vi "Reset hour counter.vi"(8 "error in (no error)":errorcluster, 10 "Button - Reset hour counter":bool, 11 "Frame Signal Conversion in":refnum<class "Frame Signal Conversion.lvclass">) -> (0 "error out":errorcluster, 3 "Frame Signal Conversion out":refnum<class "Frame Signal Conversion.lvclass">)   [LabVIEW 2024]
uses:
  Frame Signal Conversion Version 8 2015/Frame Signal Conversion Version 8/Frame Signal Conversion.lvclass
  <instrlib>/KDI Digital Instrumentation/API_for_PCAN_BASIC_FD/TPCANHandle.ctl
  Frame Signal Conversion Version 8 2015/Frame Signal Conversion Version 8/Signals to Frames/Convert Signals to Frames [Doubles].vi
  ZeroJet Test Systems/Instruments/PCAN/Polymorphic/DBC frame array to PCAN frame array.vi
  ZeroJet Test Systems/Instruments/PCAN/PCan_Xnet.lvlib
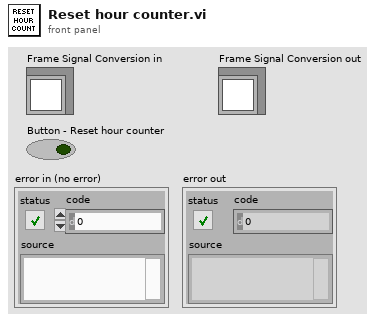
[diagram p1: front panel]
types:
  T1 = typedef "TPCANHandle.ctl" = enum16{"PCAN_NONEBUS  0x000", "PCAN_ISABUS1  0x21", "PCAN_ISABUS2  0x22", "PCAN_ISABUS3  0x23", "PCAN_ISABUS4  0x24", "PCAN_ISABUS5  0x25", "PCAN_ISABUS6  0x26", "PCAN_ISABUS7  0x27", "PCAN_ISABUS8  0x28", "PCAN_DNGBUS1  0x31", "PCAN_PCIBUS1  0x41", "PCAN_PCIBUS1  0x42", "PCAN_PCIBUS1  0x43", "PCAN_PCIBUS1  0x44", "PCAN_PCIBUS1  0x45", "PCAN_PCIBUS1  0x46", "PCAN_PCIBUS1  0x47", "PCAN_PCIBUS1  0x48", "PCAN_PCIBUS1  0x409", "PCAN_PCIBUS1  0x40A", "PCAN_PCIBUS1  0x40B", "PCAN_PCIBUS1  0x40C", "PCAN_PCIBUS1  0x40D", "PCAN_PCIBUS1  0x40E", "PCAN_PCIBUS1  0x40F", "PCAN_PCIBUS1  0x410", "PCAN_USBBUS1  0x51", "PCAN_USBBUS2  0x52", "PCAN_USBBUS3  0x53", "PCAN_USBBUS4  0x54", "PCAN_USBBUS5  0x55", "PCAN_USBBUS6  0x56", "PCAN_USBBUS7  0x57", "PCAN_USBBUS8  0x58", "PCAN_USBBUS9  0x509", "PCAN_USBBUS10  0x50A", "PCAN_USBBUS11  0x50B", "PCAN_USBBUS12  0x50C", "PCAN_USBBUS13  0x50D", "PCAN_USBBUS14  0x50E", "PCAN_USBBUS15  0x50F", "PCAN_USBBUS16  0x510", "PCAN_PCCBUS1  0x61", "PCAN_PCCBUS2  0x62", "PCAN_LANBUS1  0x801", "PCAN_LANBUS2  0x802", "PCAN_LANBUS3  0x803", "PCAN_LANBUS4  0x804", "PCAN_LANBUS5  0x805", "PCAN_LANBUS6  0x806", "PCAN_LANBUS7  0x807", "PCAN_LANBUS8  0x808", "PCAN_LANBUS9  0x809", "PCAN_LANBUS10  0x80A", "PCAN_LANBUS11  0x80B", "PCAN_LANBUS12  0x80C", "PCAN_LANBUS13  0x80D", "PCAN_LANBUS14  0x80E", "PCAN_LANBUS15  0x80F", "PCAN_LANBUS16  0x810"}
  T2 = typedef "CAN Frame XNET Model.ctl" = cluster{"timestamp":timestamp, "payload":u8[], "identifier":u32, "type":T3, "extended?":bool, "echo?":bool}
  T3 = typedef "CAN Frame Type XNET Model.ctl" = u8
  T4 = typedef "CAN MSG Cluster.ctl" = cluster{"ID":u32, "MSG type":u8, "DLC":u8, "DATA":u8[]}
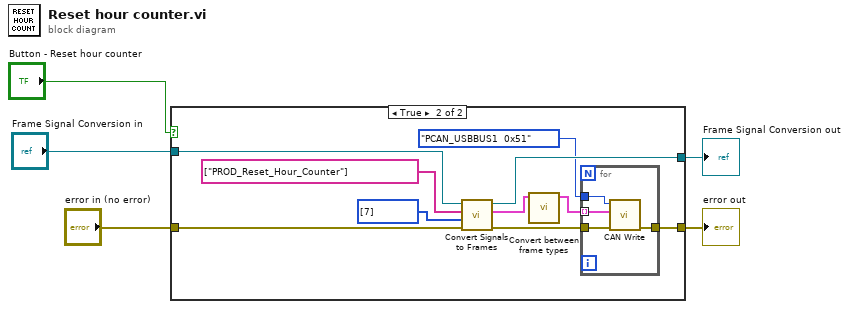
[diagram p0: block diagram]
diagram:
  n1 = case shown="True" "Button - Reset hour counter" {
    tunnel: "Frame Signal Conversion in" -> [w7 w15]
    tunnel: [w7 w14] -> w5
    tunnel: [w6 w9] -> w1
    tunnel: "error in (no error)" -> [w6 w8]
    frame False {
    }
    frame True {
      n2 = call-poly "Convert Signals to Frames.vi"("error in (no error)"=w8, "Values"=u8[] [7], "Signals"=string[] ["PROD_Reset_Hour_Counter"], "Frame Signal Conversion in"=w15) -> ("error out"=w10:errorcluster, "Frames"=w13:T2[], "Frame Signal Conversion out"=w14:refnum<class "Frame Signal Conversion.lvclass">)  [unwired: 5 in]
      n3 = call-poly "Convert between frame types.vi"("Frame input"=w13) -> ("Frame output"=w12:T4[])  [unwired: 10 in]
      n4 = for {
        tunnel: w12 -> [w21] mode=indexing
        tunnel: TPCANHandle."PCAN_USBBUS1  0x51" ("TPCANHandle") -> [w20]
        tunnel: w10 -> [w19]
        tunnel: [w18] -> w9
        n5 = call <instrlib>:"CAN Write.vi"("error in (no error)"=w19, "CAN_Message"=w21, "TPCANHandle"=w20) -> ("error out"=w18:errorcluster)  [unwired: 7 in, 1 out]
      }
    }
  }
  "Frame Signal Conversion out" <- w5
  "error out" <- w1
